vi "Huskie_RotateLEDs.vi"(7 "HBDevRef":T1, 8 "LEDs per Color":dbl=1.0, 9 "Number of LEDs":dbl, 10 "Iterations":dbl, 11 "Colors In":u32[](array[colorbox])=[16484864, 16860]) -> ()   [LabVIEW 2018]
uses:
  <vilib>/Rock Robotics/WPI/SerialPort/WPI_SerialPortRef.ctl
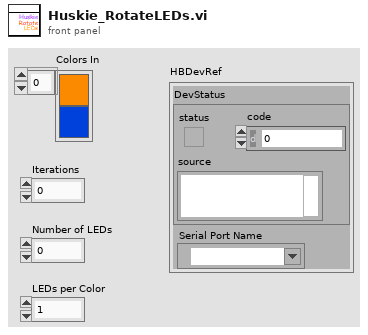
[diagram p1: front panel]
types:
  T1 = typedef "WPI_SerialPortRef.ctl" = cluster{"DevStatus":errorcluster, "Serial Port Name":refnum<visa-resource-name>}
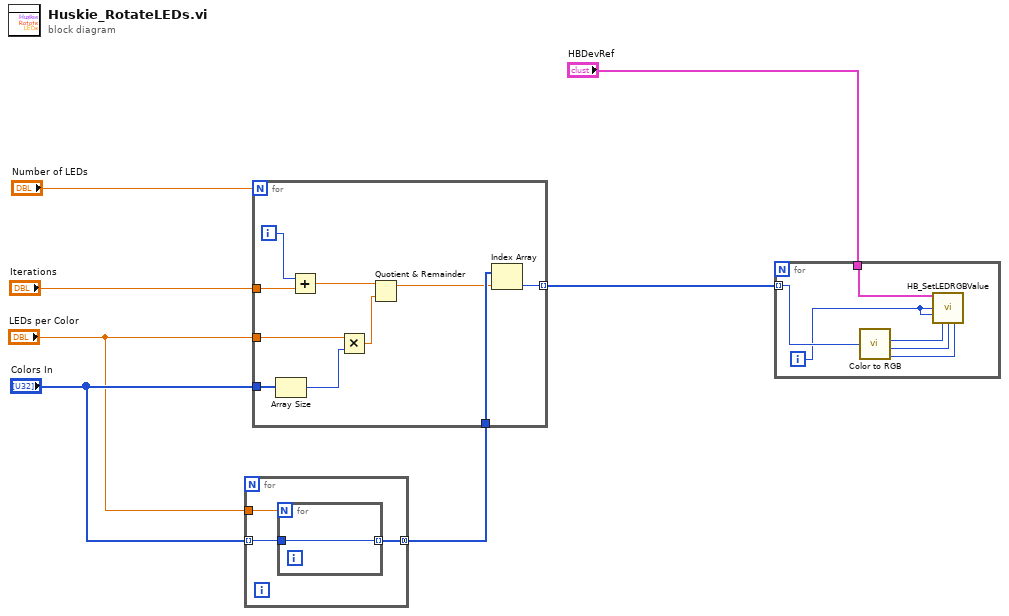
[diagram p0: block diagram]
diagram:
  n1 = for {
    tunnel: "Colors In" -> [w9] mode=indexing
    tunnel: "LEDs per Color" -> [w10]
    tunnel: [w8] -> w3 mode=concatenating
    n2 = for {
      N: w10 -> [_]
      tunnel: w9 -> [w11]
      tunnel: [w11] -> w8 mode=indexing
    }
  }
  n3 = for {
    N: "Number of LEDs" -> [_]
    tunnel: "Iterations" -> [w20]
    tunnel: [w19] -> w2 mode=indexing
    tunnel: "Colors In" -> [w18]
    tunnel: "LEDs per Color" -> [w14]
    tunnel: w3 -> [w13]
    i -> [w21]
    n4 = Array Size(array=w18) -> (size(s)=w16:i32)
    n5 = Add(x=w21, y=w20) -> (x+y=w17:dbl)
    n6 = Multiply(x=w14, y=w16) -> (x*y=w15:dbl)
    n7 = Quotient & Remainder(x=w17, y=w15) -> (x-y*floor(x/y)=w12:dbl)  [unwired: 1 out]
    n8 = Index Array(array=w13, index=w12) -> (element=w19:u32)
  }
  n9 = for {
    tunnel: w2 -> [w27] mode=indexing
    tunnel: "HBDevRef" -> [w22]
    i -> [w26]
    n10 = call <vilib>:"Color to RGB.vi"("Color"=w27) -> ("R"=w23:u8, "G"=w24:u8, "B"=w25:u8)  [unwired: 1 out]
    n11 = call <vilib>:"HB_SetLEDRGBValue.vi"("HBDevRef"=w22, "Start Channel"=w26, "End Channel"=w26, "Red"=w23, "Green"=w24, "Blue"=w25) -> ()  [unwired: 8 in, 2 out]
  }
